vi "d1000 in bit.vi"(11 "BitNo":i16) -> (3 "function return":u32)   [LabVIEW 2019, in "Dmc1000.lvlib"]
doc: "DMC1000_API DWORD WINAPI d1000_in_bit(short BitNo);"
uses:
  Dmc1000.lvlib
  Dmc1000.dll
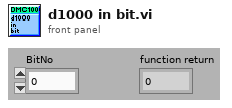
[diagram p1: front panel]
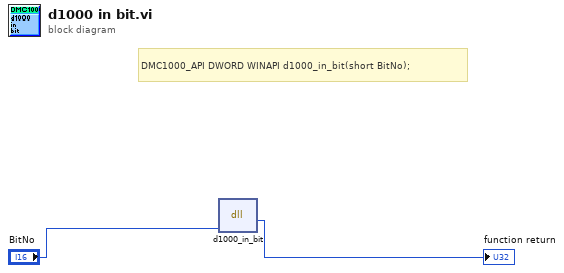
[diagram p0: block diagram]
diagram:
  # "DMC1000_API DWORD WINAPI d1000_in_bit(short BitNo);"
  n1 = dll-call lib="C:/Users/VIC/Desktop/Standar Program/System/LLB/DMC1000B/Dmc1000.*" fn="d1000_in_bit"("BitNo"="BitNo") -> (→"function return":u32)  [unwired: 4 in, 2 out]
